vi "TCP-IP Mgr.Core.vi"(10 "Q Message Templates":T3={"Status.Q.Msg"={"Cmd"="Task", "Sub"="TCP-IP Connect Event", "Data1"=variant, "Data2"=variant}, "Rcv.Q.Msg"={"Cmd"="Task", "Sub"="TCP-IP Rcv", "Data1"=variant, "Data2"=variant}}, 11 "Module Config":T1={"Name"="TCPIP_Listener", "Parent Q"=refnum, "Is Child?"=FALSE, "Index"=0, "Dirs"={"Root"=path "", "Config"=path "", "Logs"=path "", "Reports"=path "", "App Data"=path ""}, "Simulate"=FALSE}) -> ()   [LabVIEW 2017, in "TCP-IP Mgr.lvlib"]
uses:
  TCP-IP Mgr.lvlib
  <vilib>/KATE/Module/Module Config.ctl
  <vilib>/KATE/Queues/Q.Element.ctl
  <vilib>/KATE/Module/Module.Working Dirs.ctl
  TCP-IP Mgr.Cluster - Q Message Templates.ctl
  TCP-IP Mgr.Config.ctl
  <vilib>/KATE/Module/Window/Window.Task, Action.ctl
  <vilib>/KATE/Queues/Queue Utils.lvlib
  <vilib>/KATE/Module/Module Utils.lvlib
  <vilib>/KATE/Controls/Controls.lvlib
  <vilib>/KATE/Event Log/Event Log.lvlib
  <vilib>/KATE/Status/Status Utils.lvlib
panel:
  in  "Main Tab":enum32{"Operate", "Maint"}(tab)
  out "Status":string
  in  "Auto Scroll":bool
  out "Log":string
  in  "Clear":bool
  in  "Maint":bool
  out "Port":u16=8500
  in  "Show Block Diagram":bool
  in  "Leave Maint":bool
  in  "Exit":bool
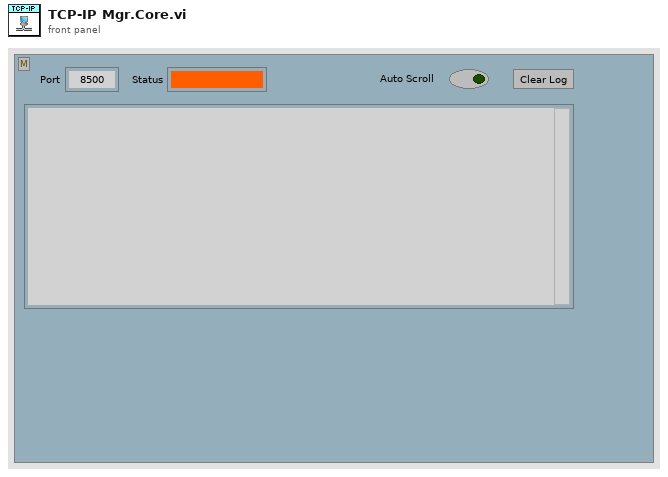
[diagram p1: front panel]
types:
  T1 = typedef "KATE_Lib.lvlib/Module Utils.lvlib/Module Config.ctl" = cluster{"Name":string, "Parent Q":refnum<queue>, "Is Child?":bool, "Index":i32, "Dirs":T2, "Simulate":bool}
  T2 = typedef "KATE_Lib.lvlib/Module Utils.lvlib/Module.Working Dirs.ctl" = cluster{"Root":path, "Config":path, "Logs":path, "Reports":path, "App Data":path}
  T3 = typedef "TCP-IP Mgr.lvlib/TCP-IP Mgr.Cluster - Q Message Templates.ctl" = cluster{"Status.Q.Msg":T4, "Rcv.Q.Msg":T4}
  T4 = typedef "KATE_Lib.lvlib/Queue Utils.lvlib/Q.Element.ctl" = cluster{"Cmd":string, "Sub":string, "Data1":variant, "Data2":variant}
  T5 = typedef "KATE_Lib.lvlib/Module Utils.lvlib/Module Sys Info.ctl" = cluster{"Main Q":refnum<queue>, "Exe":bool, "SW Rev":T6, "Self Ref":refnum<vi>, "Main Tab":refnum<vi>, "Pane":refnum<vi>, "Stop":cluster{"Ref":refnum<event-registration>, "Event":refnum<user-event>}, "Cfg":T1, "Services":cluster{"Name":string, "vi ref":refnum<vi>}[], "Menu Ref":refnum<k9>, "CtrlStates":refnum<class "Class.SaveCtrls.lvclass">, "Docs":cluster{"Tags":string[], "Paths":path[]}}
  T6 = typedef "KATE_Lib.lvlib/Module Utils.lvlib/Module.SW Version Info.ctl" = cluster{"AppName":string, "Company":string, "Version":string, "Description":string}
  T7 = typedef "KATE_Lib.lvlib/Module Utils.lvlib/Window.Task, Action.ctl" = enum16{"Resize()", "Show Panel(Bool)", "Show Scroll Bars(Bool)", "Dock to SubPanel(SubPanel Ref)", "Undock from SubPanel()", "Return to SubPanel()", "Go To Maint Tab()", "Show Maint Tab(Bool)", "Open Block Diagram()"}
  T8 = enum16{"Top Left", "Top Right", "Bottom Left", "Bottom Right"}
  T9 = typedef "KATE_Lib.lvlib/Status Utils.lvlib/Status.ErrorAction - Exit, Reset, Ignore.ctl" = enum16{"Exit", "Reset", "Ignore"}
  T10 = typedef "TCP-IP Mgr.lvlib/TCP-IP Mgr.Config.ctl" = cluster{"IP":string, "Port":u16, "Dir":bool}
  T11 = cluster{"Connected":bool, "TCPIP ID":refnum<k5>, "Config":T10, "QMsgs":T3}
  T12 = typedef "Main Q Element.ctl" = cluster{"Cmd":string, "Sub":string, "Data1":variant, "Data2":variant}
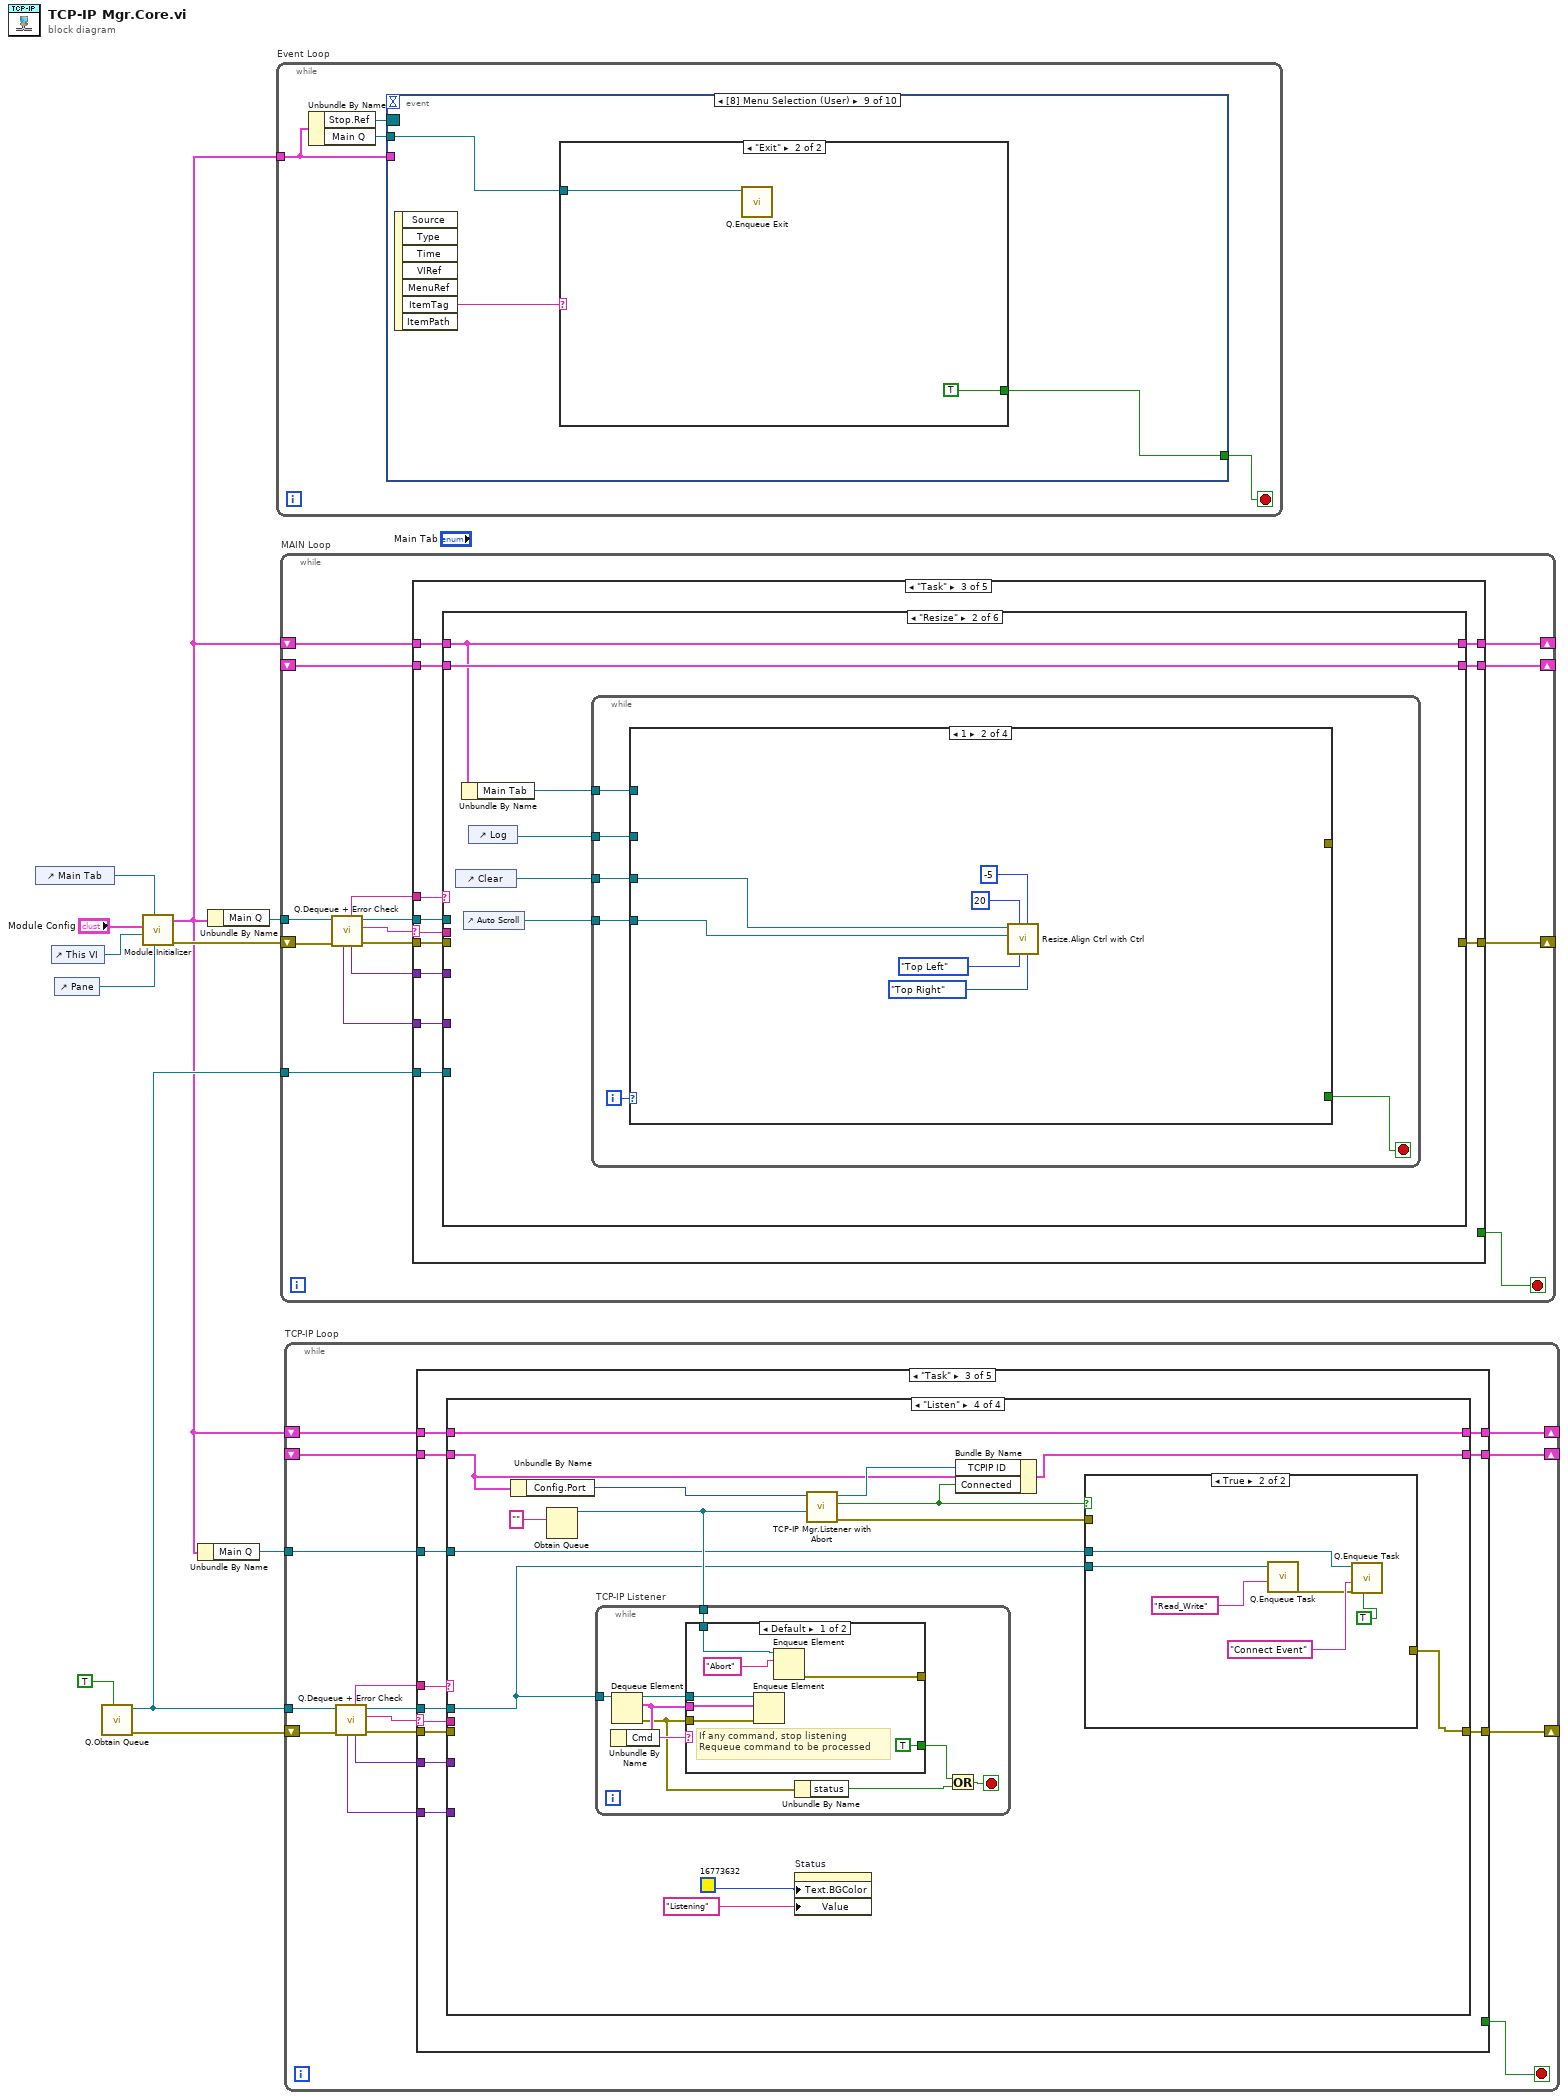
[diagram p0: block diagram]
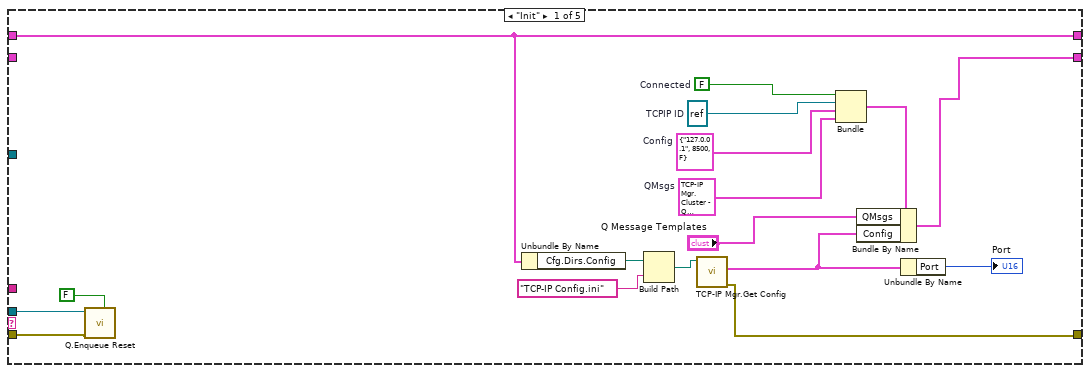
[diagram p2: hidden frame]
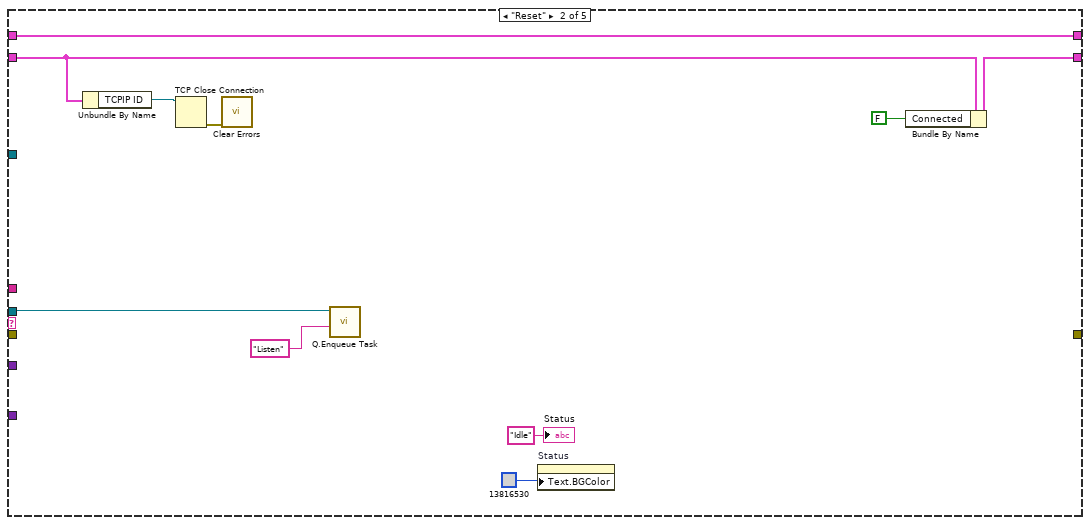
[diagram p3: hidden frame]
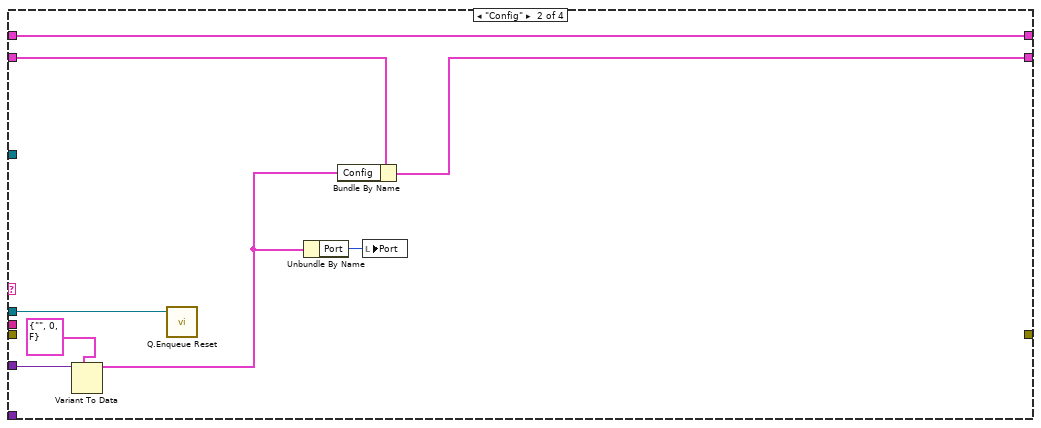
[diagram p5: hidden frame]
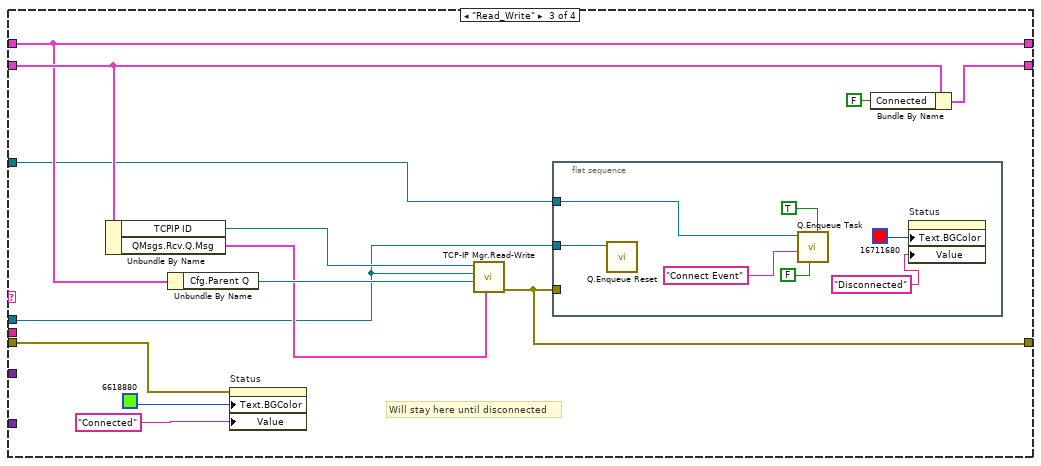
[diagram p6: hidden frame]
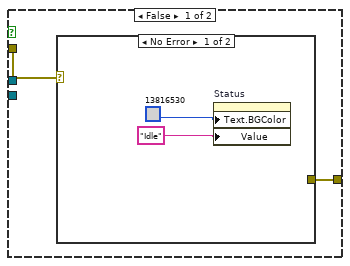
[diagram p7: hidden frame]
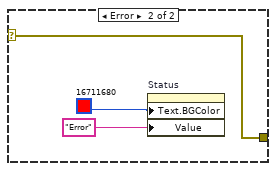
[diagram p8: hidden frame]
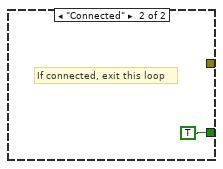
[diagram p9: hidden frame]
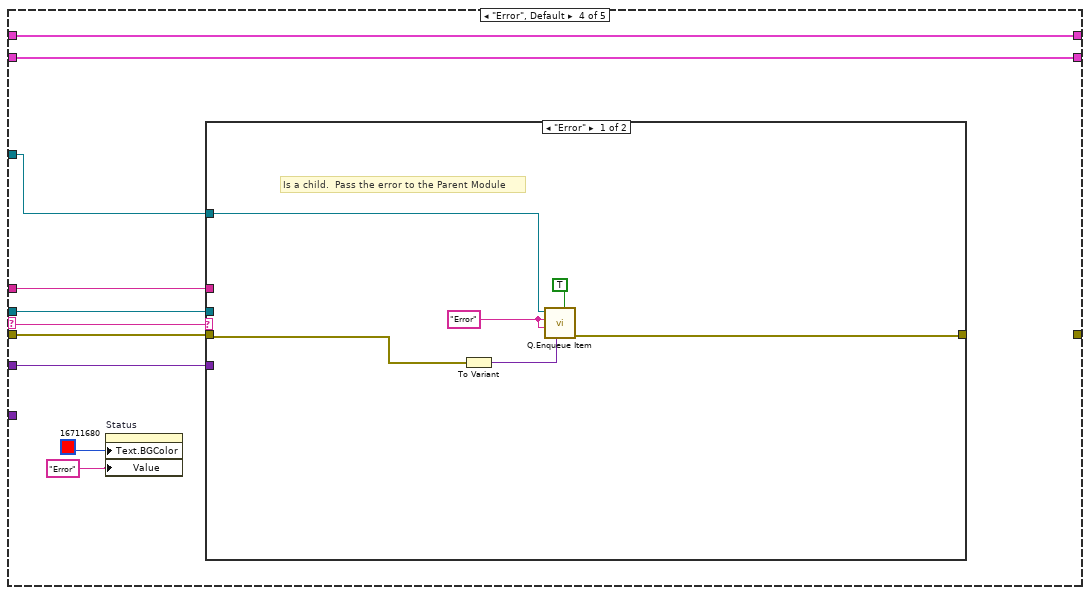
[diagram p10: hidden frame]
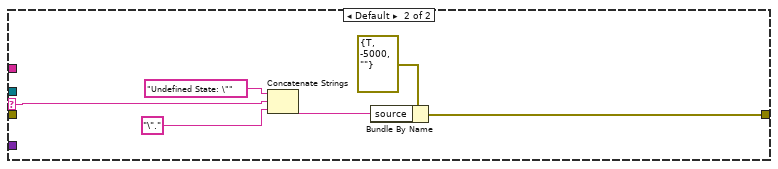
[diagram p11: hidden frame]
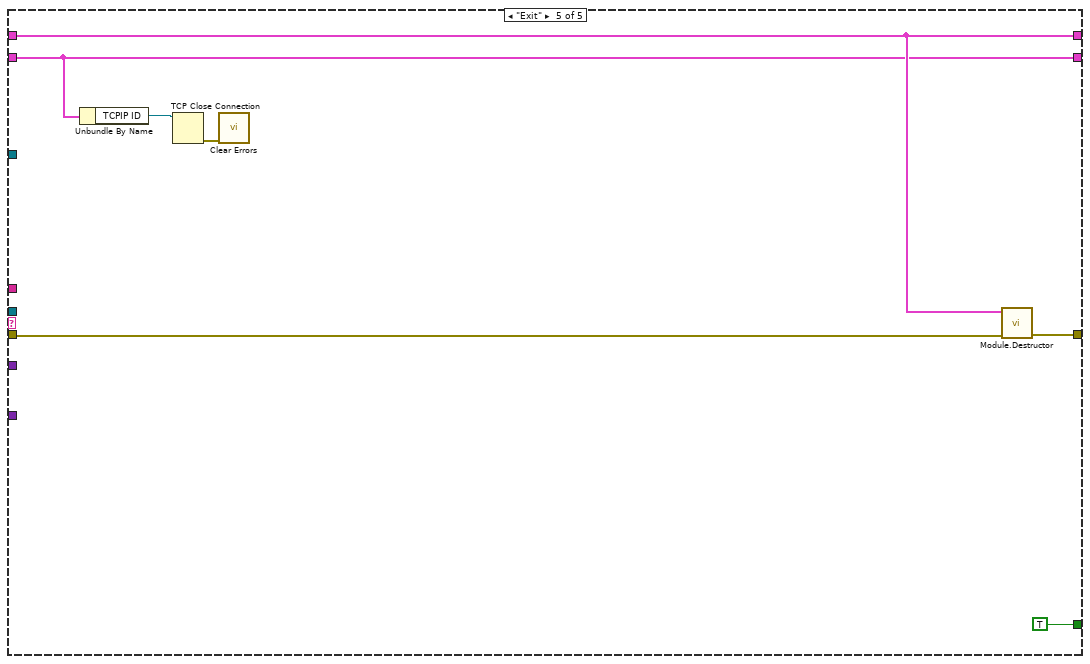
[diagram p12: hidden frame]
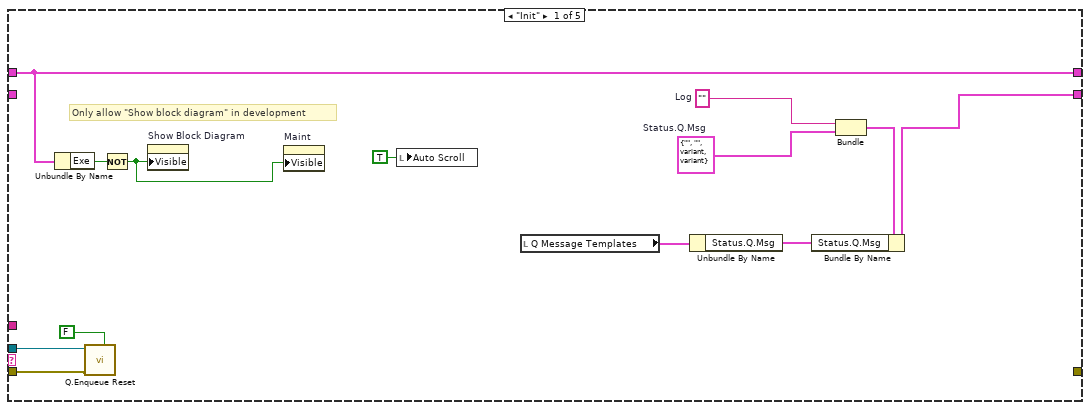
[diagram p13: hidden frame]
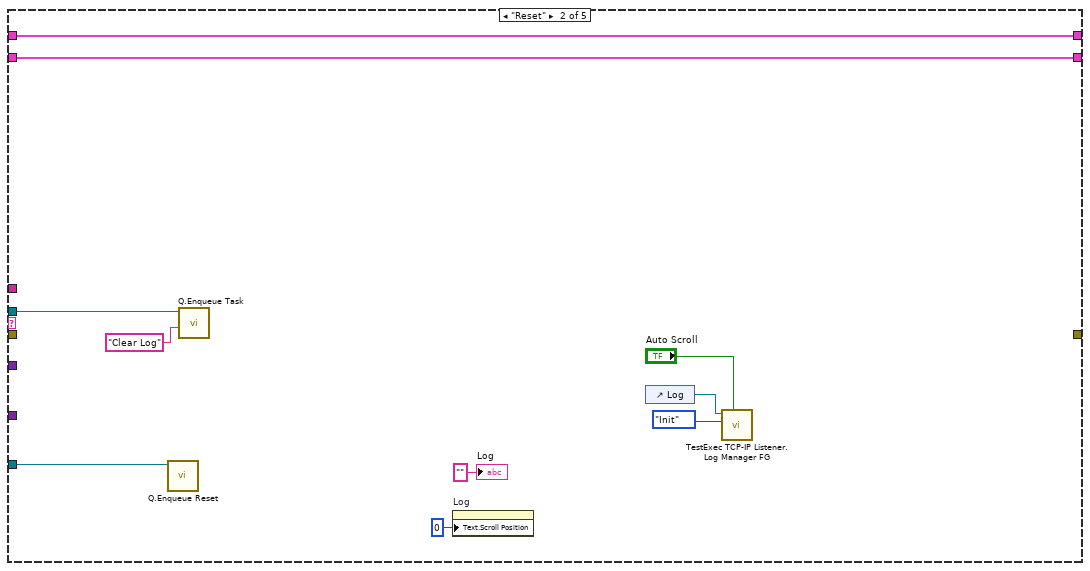
[diagram p14: hidden frame]
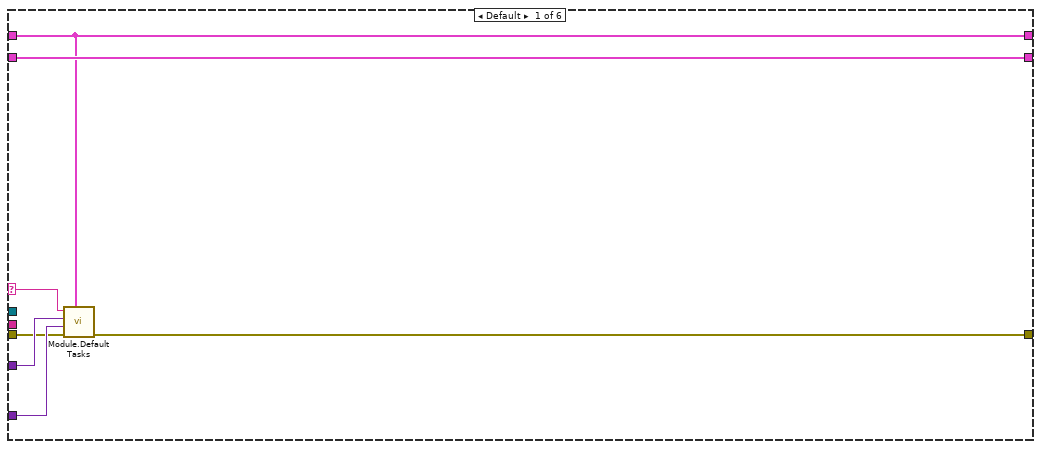
[diagram p15: hidden frame]
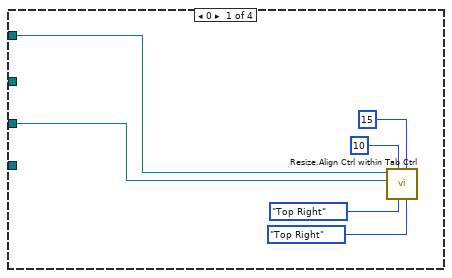
[diagram p16: hidden frame]
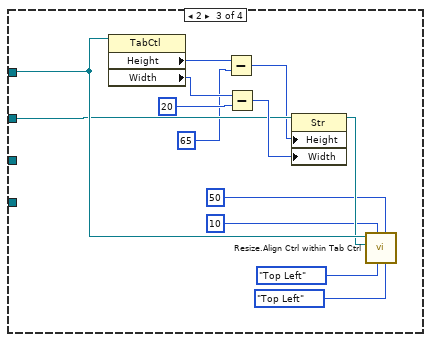
[diagram p17: hidden frame]
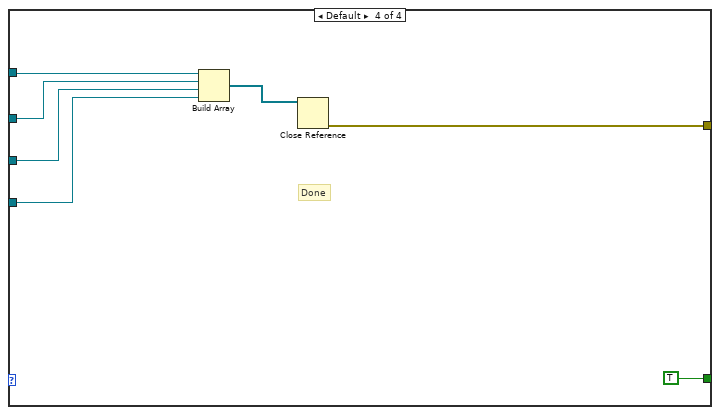
[diagram p18: hidden frame]
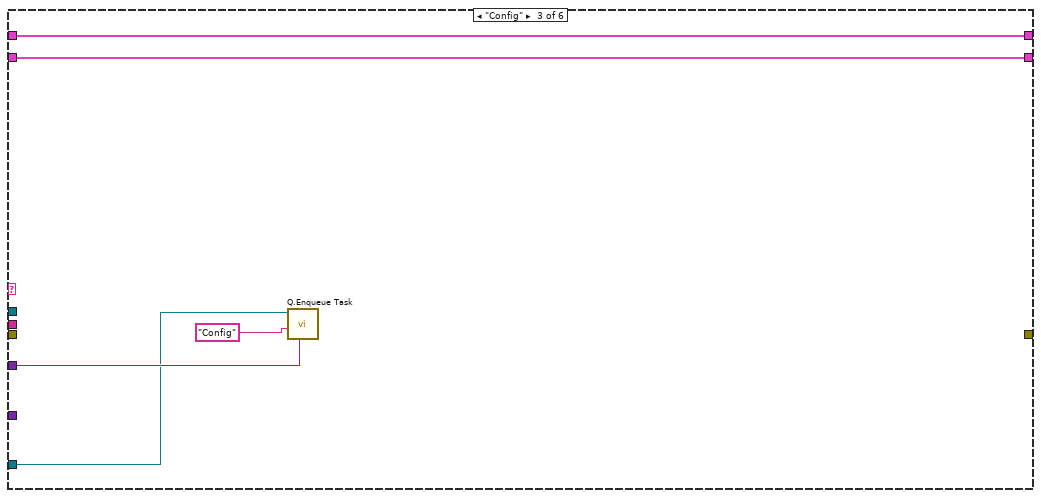
[diagram p19: hidden frame]
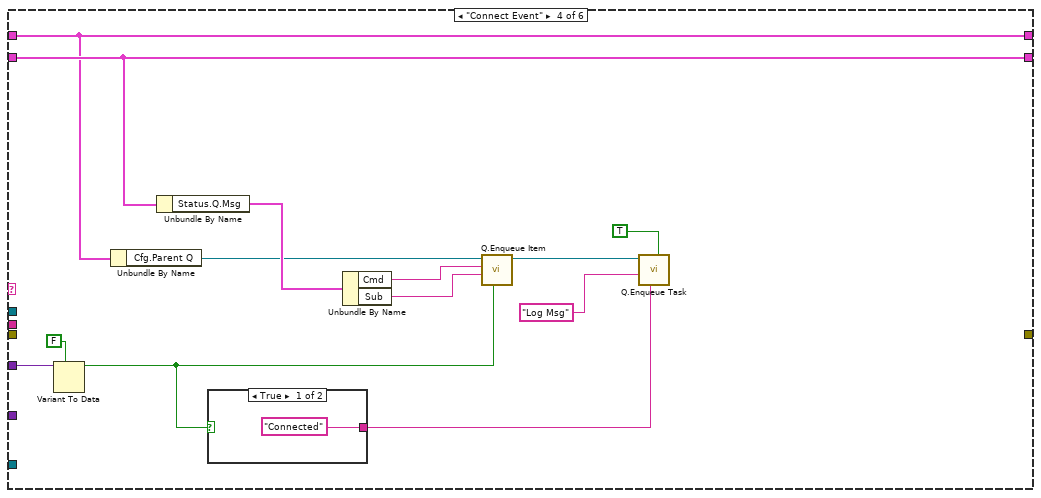
[diagram p20: hidden frame]
diagram:
  n1 = control-ref of="Main Tab"() -> (w8:refnum<vi>)
  n2 = control-ref of="This VI"() -> (w7:refnum<vi>)
  n3 = control-ref of="Pane"() -> (w6:refnum<vi>)
  n4 = call <vilib>:"Q.Obtain Queue.vi"("Enqueue Init"=TRUE) -> ("error out"=w3:errorcluster, "Q Out"=w4:refnum<queue>)  [unwired: 8 in, 1 out]
  n5 = call <vilib>:"Module.Initializer.vi"("Pane"=w6, "Main Tab"=w8, "Self Ref"=w7, "Module Config"="Module Config") -> ("error out"=w10:errorcluster, "Sys"=w1:T5)  [unwired: 6 in]
  n6 = Unbundle By Name(w1) -> ("Main Q"=w2:refnum<queue>)
  n7 = Unbundle By Name(w1) -> ("Main Q"=w9:refnum<queue>)
  n8 = while "Event Loop" {
    tunnel: w1 -> [w14]
    stop <- w15 stop-if-true
    n9 = Unbundle By Name(w14) -> ("Stop.Ref"=w13:refnum<event-registration>, "Main Q"=w12:refnum<queue>)
    n10 = event shown="[8] Menu Selection (User)" {
      selector: w13 -> [_ _ _ _ _ _ _ _ _ _]
      dyn-events: _ -> [_ _ _ _ _ _ _ _ _ _]
      timeout: _ -> [_ _ _ _ _ _ _ _ _ _]
      tunnel: [w18 _ _ _ _ _ TRUE _ w43 TRUE] -> w15
      tunnel: w14 -> [w17 _ _ _ _ _ _ _ _ _]
      tunnel: w12 -> [w20 w30 w32 w34 _ w38 w39 _ w42 _]
      event Panel Close? {
        n11 = event-data() -> ()  [unwired: 1 in, 4 out]
        n12 = Unbundle By Name(w17) -> ("Cfg.Is Child?"=w16:bool)
        n13 = case shown="False" w16 {
          tunnel: w20 -> [w23 w26]
          tunnel: [TRUE TRUE] -> w19
          tunnel: [TRUE FALSE] -> w18
          tunnel: [_ w24] -> _
          frame False {
            # "Parent - Exit"
            n14 = call <vilib>:"Q.Enqueue Exit.vi"("Q In"=w23) -> ()  [unwired: 9 in, 2 out]
          }
          frame True {
            # "Child - Hide Panel"
            n15 = call <vilib>:"Module.Window, Q Task.vi"("Action"=Window.Task,_Action."Show Panel(Bool)", "Q In"=w26) -> ("error out"=w24:errorcluster)  [unwired: 8 in, 1 out]
          }
        }
        n16 = event-data("Discard?"=w19) -> ()  [unwired: 1 in, 1 out]
      }
      event Panel Resize {
        n17 = event-data() -> ()  [unwired: 1 in, 8 out]
        n18 = call <vilib>:"Module.Window, Q Task.vi"("Action"=Window.Task,_Action."Resize()", "Q In"=w30) -> ()  [unwired: 8 in, 2 out]
      }
      event "Show Block Diagram": Value Change {
        n19 = event-data() -> ()  [unwired: 1 in, 6 out]
        n20 = call <vilib>:"Module.Window, Q Task.vi"("Action"=Window.Task,_Action."Open Block Diagram()", "Q In"=w32) -> ()  [unwired: 8 in, 2 out]
      }
      event "Maint": Value Change {
        n21 = event-data() -> ()  [unwired: 1 in, 6 out]
        n22 = call <vilib>:"Module.Window, Q Task.vi"("Action"=Window.Task,_Action."Go To Maint Tab()", "Q In"=w34) -> ()  [unwired: 8 in, 2 out]
      }
      event "Auto Scroll": Value Change {
        n23 = event-data() -> ("NewVal"=w35:bool)  [unwired: 1 in, 5 out]
        n24 = call "TestExec TCP-IP Listener.Log Manager FG.vi"("Auto Scroll"=w35, "Action"=enum16{"Init", "Clear", "Log", "Set AutoScroll"}."Set AutoScroll") -> ()  [unwired: 10 in]
      }
      event "Clear": Value Change {
        n25 = event-data() -> ()  [unwired: 1 in, 6 out]
        n26 = call <vilib>:"Q.Enqueue Task.vi"("Task Name"="Clear Log", "Q In"=w38) -> ()  [unwired: 8 in, 2 out]
      }
      event "Exit": Value Change {
        n27 = event-data() -> ()  [unwired: 1 in, 6 out]
        n28 = call <vilib>:"Q.Enqueue Exit.vi"("Q In"=w39) -> ()  [unwired: 9 in, 2 out]
      }
      event "Leave Maint": Value Change {
        n29 = event-data() -> ()  [unwired: 1 in, 6 out]
        n30 = local write "Main Tab"(0) -> ()
      }
      event Menu Selection (User) {
        n31 = event-data() -> ("ItemTag"=w44:string)  [unwired: 1 in, 6 out]
        n32 = case shown="\"Exit\"" w44 {
          tunnel: [_ TRUE] -> w43
          tunnel: w42 -> [_ w45]
          frame "False", Default {
          }
          frame "Exit" {
            n33 = call <vilib>:"Q.Enqueue Exit.vi"("Q In"=w45) -> ()  [unwired: 9 in, 2 out]
          }
        }
      }
      event User Event {
        n34 = event-data() -> ()  [unwired: 1 in, 5 out]
      }
    }
  }
  n35 = while "MAIN Loop" {
    shift-right: [w58] -> _
    shift-left: w10 -> [w56]
    shift-right: [w59] -> _
    shift-left: _ -> [w62]
    shift-right: [w60] -> _
    shift-left: w1 -> [w61]
    tunnel: w9 -> [w55]
    tunnel: w4 -> [w48]
    stop <- w49 stop-if-true
    n36 = call <vilib>:"Q.Dequeue + Error Check.vi"("Error In"=w56, "Q In"=w55) -> ("error out"=w57:errorcluster, "Cmd"=w54:string, "Q Out"=w53:refnum<queue>, "Data1"=w52:variant, "Sub"=w50:string, "Data2"=w51:variant)  [unwired: 4 in]
    n37 = case shown="\"Task\"" w54 {
      selector: w54 -> [_ _ w87 w184 _]
      tunnel: w62 -> [_ w77 w96 w189 w229]
      tunnel: w61 -> [w68 w85 w97 w181 w231]
      tunnel: [w68 w85 w95 w181 w231] -> w60
      tunnel: [w64 w77 w94 w189 w229] -> w59
      tunnel: [_ _ w88 _ w233] -> w58
      tunnel: w57 -> [w74 _ w90 w183 w232]
      tunnel: w53 -> [w75 w82 w91 w185 _]
      tunnel: w52 -> [_ _ w92 w182 _]
      tunnel: w51 -> [_ _ w89 _ _]
      tunnel: w50 -> [_ _ w93 w186 _]
      tunnel: [_ _ _ _ TRUE] -> w49
      tunnel: w48 -> [_ w76 w86 _ w228]
      frame "Init" {
        w66 = T4 {"Cmd"="", "Sub"="", "Data1"=variant, "Data2"=variant}  # Status.Q.Msg
        w69 = ""  # Log
        # "Only allow \"Show block diagram\" in development"
        n38 = Unbundle By Name(w68) -> ("Exe"=w72:bool)
        n39 = call <vilib>:"Q.Enqueue Reset.vi"("Top of Q(T)"=FALSE ("Flush Q"), "Error In"=w74, "Q In"=w75) -> ()  [unwired: 7 in, 2 out]
        n40 = Not(x=w72) -> (.not. x?=w71:bool)
        n41 = property on="Show Block Diagram" class="Bool"("Visible"=w71) -> ()  [unwired: 2 in, 2 out]
        n42 = property on="Maint" class="Bool"("Visible"=w71) -> ()  [unwired: 2 in, 2 out]
        n43 = local write "Auto Scroll"(TRUE ("Auto Scroll")) -> ()
        n44 = local read "Q Message Templates"() -> (w67:T3)
        n45 = Unbundle By Name(w67) -> ("Status.Q.Msg"=w63:T4)
        n46 = Bundle("Log"=w69, "Status.Q.Msg"=w66) -> (w65:cluster{"Log":string, "Status.Q.Msg":T4})  [unwired: 1 in]
        n47 = Bundle By Name(cluster=w65, "Status.Q.Msg"=w63) -> (w64:cluster{"Log":string, "Status.Q.Msg":T4})
      }
      frame "Reset" {
        n48 = call <vilib>:"Q.Enqueue Reset.vi"("Q In"=w76) -> ()  [unwired: 9 in, 2 out]
        n49 = call <vilib>:"Q.Enqueue Task.vi"("Task Name"="Clear Log", "Q In"=w82) -> ()  [unwired: 8 in, 2 out]
        n50 = property on="Log" class="Str"("Text.Scroll Position"=u32 0) -> ()  [unwired: 2 in, 2 out]
        n51 = control-ref of="Log"() -> (w79:refnum<vi>)
        n52 = call "TestExec TCP-IP Listener.Log Manager FG.vi"("Auto Scroll"="Auto Scroll", "Action"=enum16{"Init", "Clear", "Log", "Set AutoScroll"}."Init", "Log"=w79) -> ()  [unwired: 9 in]
        "Log" <- "" ("Log")
      }
      frame "Task" {
        n53 = case shown="\"Resize\"" w93 {
          selector: w93 -> [w102 _ _ _ _ _]
          tunnel: w97 -> [w103 w109 w153 w160 w174 w178]
          tunnel: w96 -> [w104 w110 w152 w162 w169 w177]
          tunnel: [w103 w109 w153 w160 w174 w178] -> w95
          tunnel: [w104 w110 w152 w162 w169 w177] -> w94
          tunnel: w92 -> [w101 _ w151 w163 w172 _]
          tunnel: w91 -> [_ _ _ _ _ _]
          tunnel: w90 -> [w99 _ _ _ _ _]
          tunnel: w89 -> [w100 _ _ _ _ _]
          tunnel: [w98 _ _ _ _ _] -> w88
          tunnel: w87 -> [_ _ _ _ _ _]
          tunnel: w86 -> [_ _ w150 _ _ _]
          frame Default {
            n54 = call <vilib>:"Module.Default Tasks.vi"("Sys"=w103, "error in"=w99, "Data2"=w100, "Data1"=w101, "Sub"=w102) -> ("error out"=w98:errorcluster)  [unwired: 6 in]
          }
          frame "Resize" {
            n55 = control-ref of="Clear"() -> (w106:refnum<vi>)
            n56 = Unbundle By Name(w109) -> ("Main Tab"=w108:refnum<vi>)
            n57 = control-ref of="Auto Scroll"() -> (w105:refnum<vi>)
            n58 = control-ref of="Log"() -> (w107:refnum<vi>)
            n59 = while {
              tunnel: w108 -> [w114]
              tunnel: w107 -> [w113]
              tunnel: w106 -> [w112]
              tunnel: w105 -> [w111]
              i -> [w116]
              stop <- w115 stop-if-true
              n60 = case shown="1" w116 {
                tunnel: [_ _ _ TRUE] -> w115
                tunnel: w114 -> [w120 _ w139 w147]
                tunnel: w113 -> [_ _ w133 w146]
                tunnel: w112 -> [w118 w124 _ w145]
                tunnel: w111 -> [_ w123 _ w144]
                tunnel: [_ _ _ w142] -> _
                frame 0 {
                  n61 = call <vilib>:"Resize.Align Ctrl within Tab Ctrl.vi"("Child Ref Pos"=T8."Top Right", "dY"=15 ("dX"), "Parent Ref Pos"=T8."Top Right", "dX"=10, "Child Ctrl"=w118, "Parent Tab Ctrl"=w120) -> ()  [unwired: 3 in, 3 out]
                }
                frame 1 {
                  n62 = call <vilib>:"Resize.Align Ctrl with Ctrl.vi"("Move Ctrl Ref Location"=T8."Top Right" ("Child Ref Pos"), "dY"=-5 ("dX"), "Ref Ctrl Corner"=T8."Top Left" ("Parent Ref Pos"), "dX"=20, "Move Ctrl"=w123, "Ref Ctrl"=w124) -> ()  [unwired: 3 in, 3 out]
                }
                frame 2 {
                  n63 = property class="TabCtl"(reference=w139) -> ("Height"=w138:u32, "Width"=w137:u32)  [unwired: 1 in, 2 out]
                  n64 = Subtract(x=w138, y=u32 65) -> (x-y=w129:u32)
                  n65 = Subtract(x=w137, y=u32 20) -> (x-y=w135:u32)
                  n66 = property class="Str"(reference=w133, "Height"=w129, "Width"=w135) -> (reference out=w134:refnum<vi>)  [unwired: 1 in, 1 out]
                  n67 = call <vilib>:"Resize.Align Ctrl within Tab Ctrl.vi"("Child Ref Pos"=T8."Top Left", "dY"=u32 50 ("y"), "Parent Ref Pos"=T8."Top Left", "dX"=u32 10 ("y"), "Child Ctrl"=w134, "Parent Tab Ctrl"=w139) -> ()  [unwired: 3 in, 3 out]
                }
                frame Default {
                  # "Done"
                  n68 = Build Array(w147, w146, w145, w144) -> (w143:refnum<vi>[])
                  n69 = Close Reference(reference=w143) -> (error out=w142:errorcluster)  [unwired: 1 in]
                }
              }
            }
          }
          frame "Config" {
            n70 = call <vilib>:"Q.Enqueue Task.vi"("Data1"=w151, "Task Name"="Config", "Q In"=w150) -> ()  [unwired: 7 in, 2 out]
          }
          frame "Connect Event" {
            n71 = Variant To Data(type=FALSE, Variant=w163) -> (data=w158:bool)  [unwired: 1 in, 1 out]
            n72 = Unbundle By Name(w160) -> ("Cfg.Parent Q"=w159:refnum<queue>)
            n73 = Unbundle By Name(w162) -> ("Status.Q.Msg"=w161:T4)
            n74 = case shown="True" w158 {
              tunnel: ["Connected" ("Status") "Disconnected" ("Status")] -> w154
              frame True {
              }
              frame False {
              }
            }
            n75 = Unbundle By Name(w161) -> ("Cmd"=w165:string, "Sub"=w164:string)
            n76 = call <vilib>:"Q.Enqueue Item.vi"("Data1"=w158, "Sub"=w164, "Cmd"=w165, "Q In"=w159) -> ("Q Out"=w156:refnum<queue>)  [unwired: 6 in, 1 out]
            n77 = call <vilib>:"Q.Enqueue Task.vi"("Top of Q"=TRUE, "Data1"=w154, "Task Name"="Log Msg", "Q In"=w156) -> ()  [unwired: 6 in, 2 out]
          }
          frame "Log Msg" {
            n78 = Variant To Data(type="", Variant=w172) -> (data=w171:string)  [unwired: 1 in, 1 out]
            n79 = call "TestExec TCP-IP Listener.Log Manager FG.vi"("Data"=w171, "Action"=enum16{"Init", "Clear", "Log", "Set AutoScroll"}."Log") -> ()  [unwired: 10 in]
          }
          frame "Clear Log" {
            n80 = invoke on="Log" class="Str" method="Reinit To Default"() -> ()  [unwired: 3 in, 3 out]
            n81 = call "TestExec TCP-IP Listener.Log Manager FG.vi"("Action"=enum16{"Init", "Clear", "Log", "Set AutoScroll"}."Clear") -> ()  [unwired: 11 in]
            n82 = property on="Log" class="Str"("Text.Scroll Position"=u32 0) -> ()  [unwired: 2 in, 2 out]
          }
        }
      }
      frame "Error", Default {
        n83 = Unbundle By Name(w181) -> ("Cfg.Is Child?"=w188:bool, "Cfg.Parent Q"=w187:refnum<queue>)
        n84 = property on="Status" class="Str"("Text.BGColor"=u32 16711680, "Value"="Error" ("Status")) -> ()  [unwired: 2 in, 2 out]
        n85 = case shown="\"Error\"" w184 {
          selector: w184 -> [_ w222]
          tunnel: [w192 w223] -> _
          tunnel: w182 -> [w196 _]
          tunnel: w183 -> [w194 _]
          tunnel: w186 -> [w195 _]
          tunnel: w185 -> [w193 _]
          tunnel: w188 -> [w191 _]
          tunnel: w187 -> [w190 _]
          frame "Error" {
            n86 = case shown="False" w191 {
              tunnel: w196 -> [w205 _]
              tunnel: w195 -> [w204 _]
              tunnel: w194 -> [w203 w218]
              tunnel: w193 -> [w201 _]
              tunnel: [w199 w216] -> w192
              tunnel: w190 -> [_ w221]
              frame False {
                # "Is running as Parent or Individual Module\nHandle Error Here"
                n87 = case shown="\"Error\"" w204 {
                  tunnel: w205 -> [_ w215]
                  tunnel: w203 -> [w211 _]
                  tunnel: [w211 w213] -> w198
                  tunnel: w201 -> [w210 w212]
                  tunnel: [w210 w212] -> w200
                  frame Default {
                  }
                  frame "Error" {
                    n88 = Variant To Data(type=errorcluster {"status"=FALSE, "code"=0, "source"=""} ("error constant"), Variant=w215) -> (data=w213:errorcluster)  [unwired: 1 in, 1 out]
                  }
                }
                n89 = call <vilib>:"Status.Dialog - Error Message.vi"("error in"=w198) -> ("Selection"=w202:T9)
                n90 = call <vilib>:"Event Log.Record Event.vi"("error in"=w198) -> ("error out"=w197:errorcluster)  [unwired: 10 in]
                n91 = case shown="\"Exit\", Default" w202 {
                  tunnel: w200 -> [w207 _ w209]
                  tunnel: [w206 _ w208] -> w199
                  tunnel: w197 -> [_ _ _]
                  frame "Exit", Default {
                    n92 = call <vilib>:"Q.Enqueue Exit.vi"("Q In"=w207) -> ("error out"=w206:errorcluster)  [unwired: 9 in, 1 out]
                  }
                  frame "Ignore" {
                  }
                  frame "Reset" {
                    n93 = call <vilib>:"Q.Enqueue Reset.vi"("Q In"=w209) -> ("error out"=w208:errorcluster)  [unwired: 9 in, 1 out]
                  }
                }
              }
              frame True {
                w219 = "Error" ("Cmd")
                # "Is a child.  Pass the error to the Parent Module"
                n94 = To Variant(anything=w218) -> (Variant=w217:variant)
                n95 = call <vilib>:"Q.Enqueue Item.vi"("Top of Q"=TRUE, "Data1"=w217, "Sub"=w219, "Cmd"=w219, "Q In"=w221) -> ("error out"=w216:errorcluster)  [unwired: 5 in, 1 out]
              }
            }
          }
          frame Default {
            n96 = Concatenate Strings("Undefined State: \"", w222, "\".") -> (w224:string)
            n97 = Bundle By Name(cluster=errorcluster {"status"=TRUE, "code"=-5000, "source"=""} ("error constant"), "source"=w224) -> (w223:errorcluster)
          }
        }
      }
      frame "Exit" {
        n98 = call <vilib>:"Q.Enqueue Exit.vi"("Q In"=w228) -> ()  [unwired: 9 in, 2 out]
        n99 = call <vilib>:"Module.Destructor.vi"("error in"=w232, "Sys"=w231) -> ("error out"=w233:errorcluster)  [unwired: 9 in]
      }
    }
  }
  n100 = while "TCP-IP Loop" {
    shift-right: [w244] -> _
    shift-left: w3 -> [w242]
    shift-right: [w245] -> _
    shift-left: _ -> [w248]
    shift-right: [w246] -> _
    shift-left: w1 -> [w247]
    tunnel: w4 -> [w241]
    tunnel: w2 -> [w234]
    stop <- w235 stop-if-true
    n101 = call <vilib>:"Q.Dequeue + Error Check.vi"("Error In"=w242, "Q In"=w241) -> ("error out"=w243:errorcluster, "Cmd"=w240:string, "Q Out"=w239:refnum<queue>, "Data1"=w238:variant, "Sub"=w236:string, "Data2"=w237:variant)  [unwired: 4 in]
    n102 = case shown="\"Task\"" w240 {
      selector: w240 -> [_ _ w277 w368 _]
      tunnel: w248 -> [_ w273 w286 w371 w384]
      tunnel: w247 -> [w255 w275 w287 w365 w388]
      tunnel: [w255 w275 w285 w365 w388] -> w246
      tunnel: [w258 w274 w284 w371 w384] -> w245
      tunnel: [w254 _ w278 _ w390] -> w244
      tunnel: w243 -> [w264 _ w280 w367 w389]
      tunnel: w239 -> [w265 w268 w281 w369 _]
      tunnel: w238 -> [_ _ w282 w366 _]
      tunnel: w237 -> [_ _ w279 _ _]
      tunnel: w236 -> [_ _ w283 w370 _]
      tunnel: [_ _ _ _ TRUE] -> w235
      tunnel: w234 -> [_ _ w276 w362 _]
      frame "Init" {
        w256 = T3 {"Status.Q.Msg"={"Cmd"="Task", "Sub"="TCP-IP Connect Event", "Data1"=variant, "Data2"=variant}, "Rcv.Q.Msg"={"Cmd"="Task", "Sub"="TCP-IP Rcv", "Data1"=variant, "Data2"=variant}}  # QMsgs
        w260 = T10 {"IP"="127.0.0.1", "Port"=8500, "Dir"=FALSE}  # Config
        w261 = refnum<k5> refnum  # TCPIP ID
        w262 = FALSE  # Connected
        n103 = call <vilib>:"Q.Enqueue Reset.vi"("Top of Q(T)"=FALSE ("Flush Q"), "Error In"=w264, "Q In"=w265) -> ()  [unwired: 7 in, 2 out]
        n104 = Unbundle By Name(w255) -> ("Cfg.Dirs.Config"=w253:path)
        n105 = Build Path(base path=w253, name or relative path="TCP-IP Config.ini") -> (appended path=w251:path)
        n106 = call "TCP-IP Mgr.Get Config.vi"("Path"=w251) -> ("error out"=w254:errorcluster, "Config Out"=w257:T10)  [unwired: 9 in]
        n107 = Bundle("Connected"=w262, "TCPIP ID"=w261, "Config"=w260, "QMsgs"=w256) -> (w259:T11)  [unwired: 1 in]
        n108 = Bundle By Name(cluster=w259, "QMsgs"="Q Message Templates", "Config"=w257) -> (w258:T11)
        n109 = Unbundle By Name(w257) -> ("Port"=→"Port":u16)
      }
      frame "Reset" {
        n110 = Unbundle By Name(w273) -> ("TCPIP ID"=w271:refnum<k5>)
        n111 = TCP Close Connection(connection ID=w271) -> (error out=w272:errorcluster)  [unwired: 2 in, 1 out]
        n112 = call <vilib>:"Clear Errors.vi"("error in (no error)"=w272) -> ()  [unwired: 5 in, 2 out]
        n113 = call <vilib>:"Q.Enqueue Task.vi"("Task Name"="Listen", "Q In"=w268) -> ()  [unwired: 8 in, 2 out]
        n114 = property on="Status" class="Str"("Text.BGColor"=u32 13816530) -> ()  [unwired: 2 in, 2 out]
        n115 = Bundle By Name(cluster=w273, "Connected"=FALSE ("Running")) -> (w274:T11)
        "Status" <- "Idle" ("Status")
      }
      frame "Task" {
        n116 = case shown="\"Listen\"" w283 {
          tunnel: w287 -> [w288 w297 w305 w331]
          tunnel: w286 -> [w289 w292 w306 w322]
          tunnel: [w288 w297 w305 w331] -> w285
          tunnel: [w289 w291 w309 w321] -> w284
          tunnel: w282 -> [_ w293 _ _]
          tunnel: w281 -> [_ w290 w298 w323]
          tunnel: w280 -> [_ _ w301 _]
          tunnel: w279 -> [_ _ _ _]
          tunnel: [_ _ w307 w324] -> w278
          tunnel: w277 -> [_ _ _ _]
          tunnel: w276 -> [_ _ w299 w318]
          frame Default {
            # "Do Nothing"
          }
          frame "Config" {
            n117 = Variant To Data(type=T10 {"IP"="", "Port"=0, "Dir"=FALSE} ("Config"), Variant=w293) -> (data=w294:T10)  [unwired: 1 in, 1 out]
            n118 = call <vilib>:"Q.Enqueue Reset.vi"("Q In"=w290) -> ()  [unwired: 9 in, 2 out]
            n119 = Unbundle By Name(w294) -> ("Port"=w295:u16)
            n120 = Bundle By Name(cluster=w292, "Config"=w294) -> (w291:T11)
            n121 = local write "Port"(w295) -> ()
          }
          frame "Read_Write" {
            # "Will stay here until disconnected"
            n122 = Unbundle By Name(w306) -> ("TCPIP ID"=w308:refnum<k5>, "QMsgs.Rcv.Q.Msg"=w303:T4)
            n123 = Unbundle By Name(w305) -> ("Cfg.Parent Q"=w304:refnum<queue>)
            n124 = property on="Status" class="Str"(error in=w301, "Text.BGColor"=u32 6618880, "Value"="Connected" ("Status")) -> ()  [unwired: 1 in, 2 out]
            n125 = call "TCP-IP Mgr.Read-Write.vi"("Rcv Q.Element"=w303, "Q.Out"=w304, "Q In"=w298, "TCPIP ID"=w308) -> ("error out"=w307:errorcluster)  [unwired: 7 in]
            n126 = flat-sequence {
              tunnel: w299 -> [w314]
              tunnel: w307 -> [_]
              tunnel: w298 -> [w313]
              frame #0 {
                n127 = call <vilib>:"Q.Enqueue Reset.vi"("Q In"=w313) -> ()  [unwired: 9 in, 2 out]
                n128 = call <vilib>:"Q.Enqueue Task.vi"("Top of Q"=TRUE, "Data1"=FALSE, "Task Name"="Connect Event" ("Cmd"), "Q In"=w314) -> ()  [unwired: 6 in, 2 out]
                n129 = property on="Status" class="Str"("Text.BGColor"=u32 16711680, "Value"="Disconnected" ("Status")) -> ()  [unwired: 2 in, 2 out]
              }
            }
            n130 = Bundle By Name(cluster=w306, "Connected"=FALSE) -> (w309:T11)
          }
          frame "Listen" {
            n131 = Unbundle By Name(w322) -> ("Config.Port"=w328:u16)
            n132 = Obtain Queue(element data type="") -> (queue out=w329:refnum<queue>)  [unwired: 4 in, 2 out]
            n133 = while "TCP-IP Listener" {
              tunnel: w323 -> [w353]
              tunnel: w329 -> [w348]
              stop <- w351 stop-if-true
              n134 = Dequeue Element(queue=w353) -> (queue out=w347:refnum<queue>, element=w346:T12, error out=w345:errorcluster)  [unwired: 2 in, 1 out]
              n135 = Unbundle By Name(w346) -> ("Cmd"=w350:string)
              n136 = case shown="Default" w350 {
                tunnel: [TRUE TRUE] -> w349
                tunnel: w348 -> [w359 _]
                tunnel: w347 -> [w357 _]
                tunnel: w346 -> [w356 _]
                tunnel: w345 -> [w355 _]
                tunnel: [w354 _] -> _
                frame Default {
                  # "If any command, stop listening\nRequeue command to be processed"
                  n137 = Enqueue Element(queue=w357, element=w356, error in (no error)=w355) -> ()  [unwired: 1 in, 3 out]
                  n138 = Enqueue Element(queue=w359, element="Abort") -> (error out=w354:errorcluster)  [unwired: 2 in, 2 out]
                }
                frame "Connected" {
                  # "If connected, exit this loop"
                }
              }
              n139 = Unbundle By Name(w345) -> ("status"=w352:bool)
              n140 = Or(x=w349, y=w352) -> (x .or. y?=w351:bool)
            }
            n141 = property on="Status" class="Str"("Text.BGColor"=u32 16773632, "Value"="Listening" ("Status")) -> ()  [unwired: 2 in, 2 out]
            n142 = call "TCP-IP Mgr.Listener with Abort.vi"("Q.Abort"=w329, "port"=w328) -> ("error out"=w325:errorcluster, "Connected"=w326:bool, "Connection ID"=w327:refnum<k5>)  [unwired: 4 in, 3 out]
            n143 = Bundle By Name(cluster=w322, "TCPIP ID"=w327, "Connected"=w326) -> (w321:T11)
            n144 = case shown="True" w326 {
              tunnel: w323 -> [_ w342]
              tunnel: w325 -> [w333 _]
              tunnel: [w332 _] -> w324
              tunnel: w318 -> [_ w339]
              frame False {
                n145 = case shown="No Error" w333 {
                  selector: w333 -> [_ w338]
                  tunnel: [_ w338] -> w332
                  frame No Error {
                    n146 = property on="Status" class="Str"("Text.BGColor"=u32 13816530, "Value"="Idle" ("Status")) -> ()  [unwired: 2 in, 2 out]
                  }
                  frame Error {
                    n147 = property on="Status" class="Str"("Text.BGColor"=u32 16711680, "Value"="Error" ("Status")) -> ()  [unwired: 2 in, 2 out]
                  }
                }
              }
              frame True {
                n148 = call <vilib>:"Q.Enqueue Task.vi"("Task Name"="Read_Write" ("Cmd"), "Q In"=w342) -> ("error out"=w343:errorcluster)  [unwired: 8 in, 1 out]
                n149 = call <vilib>:"Q.Enqueue Task.vi"("Data1"=TRUE, "Error In"=w343, "Task Name"="Connect Event" ("Cmd"), "Q In"=w339) -> ()  [unwired: 6 in, 2 out]
              }
            }
          }
        }
      }
      frame "Error", Default {
        n150 = property on="Status" class="Str"("Text.BGColor"=u32 16711680, "Value"="Error" ("Status")) -> ()  [unwired: 2 in, 2 out]
        n151 = case shown="\"Error\"" w368 {
          selector: w368 -> [_ w378]
          tunnel: [w376 w379] -> _
          tunnel: w366 -> [_ _]
          tunnel: w367 -> [w377 _]
          tunnel: w370 -> [_ _]
          tunnel: w369 -> [_ _]
          tunnel: w362 -> [w375 _]
          frame "Error" {
            w373 = "Error" ("Cmd")
            # "Is a child.  Pass the error to the Parent Module"
            n152 = To Variant(anything=w377) -> (Variant=w372:variant)
            n153 = call <vilib>:"Q.Enqueue Item.vi"("Top of Q"=TRUE, "Data1"=w372, "Sub"=w373, "Cmd"=w373, "Q In"=w375) -> ("error out"=w376:errorcluster)  [unwired: 5 in, 1 out]
          }
          frame Default {
            n154 = Concatenate Strings("Undefined State: \"", w378, "\".") -> (w380:string)
            n155 = Bundle By Name(cluster=errorcluster {"status"=TRUE, "code"=-5000, "source"=""} ("error constant"), "source"=w380) -> (w379:errorcluster)
          }
        }
      }
      frame "Exit" {
        n156 = Unbundle By Name(w384) -> ("TCPIP ID"=w385:refnum<k5>)
        n157 = TCP Close Connection(connection ID=w385) -> (error out=w386:errorcluster)  [unwired: 2 in, 1 out]
        n158 = call <vilib>:"Clear Errors.vi"("error in (no error)"=w386) -> ()  [unwired: 5 in, 2 out]
        n159 = call <vilib>:"Module.Destructor.vi"("error in"=w389, "Sys"=w388) -> ("error out"=w390:errorcluster)  [unwired: 9 in]
      }
    }
  }
